vi "main.vi"() -> ()   [LabVIEW 2025]
uses:
  Controls/#typedef States.ctl
  Data.ctl
  <vilib>/Analysis/3filter.llb/Filter Passband Type.ctl
  <vilib>/sound2/lvsound2.llb/Sampling Mode.ctl
  <vilib>/sound2/lvsound2.llb/Sound Data Format.ctl
  <vilib>/Instr/_visa.llb/VISA Configure Serial Port (Instr).vi
  <vilib>/Analysis/3filter.llb/Butterworth Filter (DBL).vi
  <vilib>/sound2/lvsound2.llb/Sound Output Write (DBL Single).vi
  <vilib>/Analysis/NI_AALBase.lvlib
panel:
  in  "DETUNE":dbl(knob) scale=0.0..1.0
  out "zoom wave":dbl[](graph)
  in  "DRIVE":dbl(slide)=1.0 scale=0.5..5.0
  in  "NOTE":enum32{"BASS", "LOW MID", "MID", "HIGH", "LEAD"}(radio)
  in  "WAVE TYPE":u16(ring) items=["SIN", "SAW", "SQUARE", "TRIANGLE"]
  in  "PORT":refnum<visa-resource-name>
  in  "Sustain":dbl(knob) scale=0.001..1.0
  in  "CUTOFF":dbl(knob) scale=1000.0..10000.0
  in  "BITCRUSHER":dbl(knob) scale=1.0..50.0
  in  "Duration [sec]":dbl(slide) scale=0.1..1.0
  in  "Decay":dbl(knob) scale=0.0..1.0
  in  "Release":dbl(knob) scale=0.0..1.0
  in  "Attack":dbl(knob) scale=0.0..1.0
  out "synth wave":i8[](graph)
  in  "TEST":bool
  in  "TRACK":enum32{"Item 0", "Item 1", "", "  "}(radio)
  out "error out":errorcluster
  in  "error in (no error)":errorcluster
  in  "stop":bool
  in  "SEND":bool
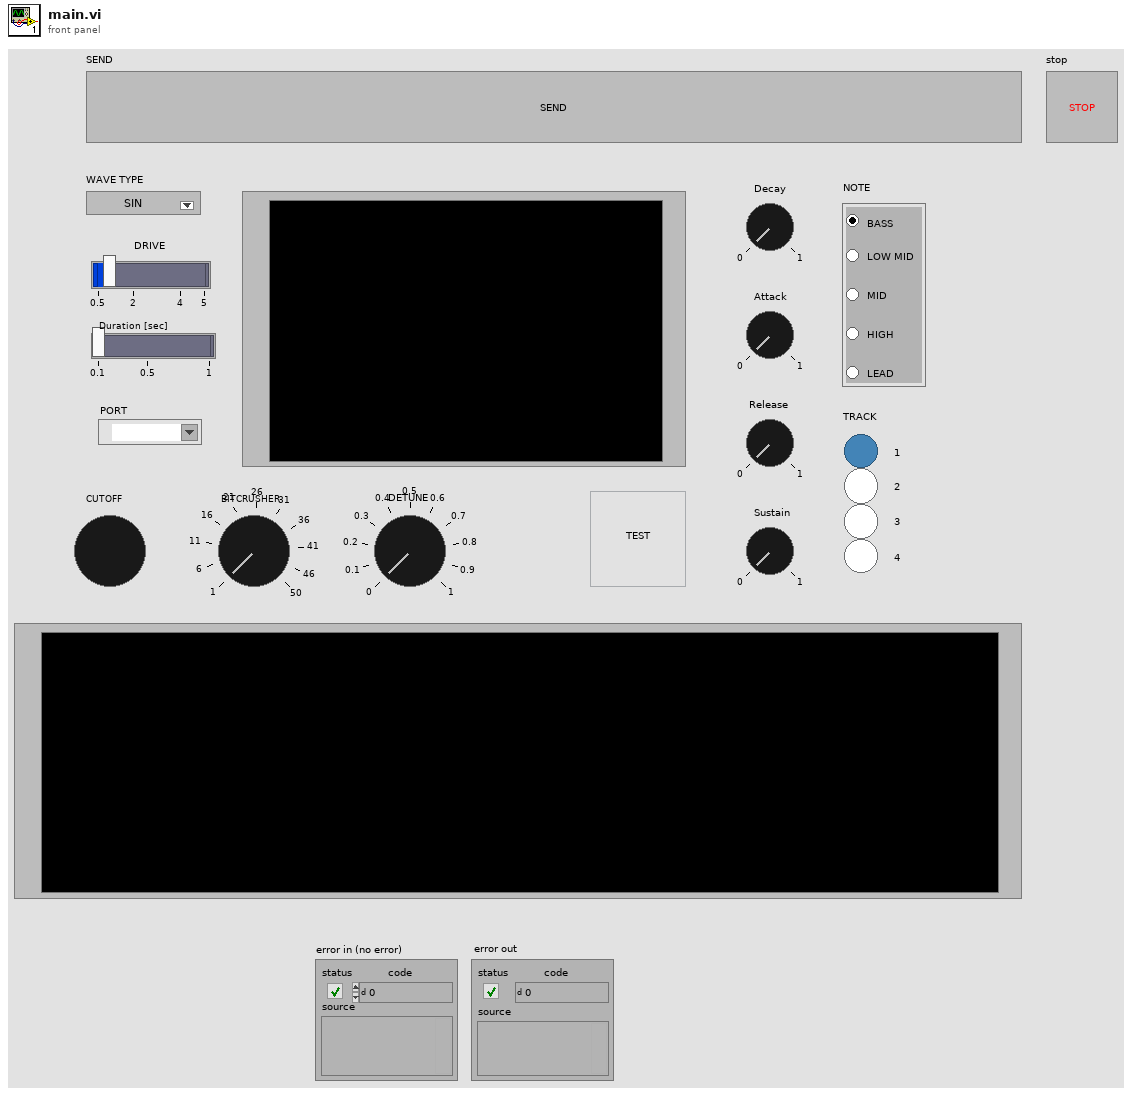
[diagram p1: front panel]
types:
  T1 = typedef "Data.ctl" = cluster{"Test/Send flag":bool, "TestData":dbl[], "8bitData":i8[], "VISA resource name":refnum<visa-resource-name>, "Decay":dbl, "Release":dbl, " Attack":dbl, "Sustain Level":dbl, "Cutoff":dbl, "Bitcrusher":dbl, "SampleLenght":dbl, "WAVE TYPE":u16, "Duration [sec]":dbl, "DRIVE":dbl, "NOTE":enum32{"BASS", "LOW MID", "MID", "HIGH", "LEAD"}, "Detune":dbl}
  T2 = typedef "#typedef States.ctl" = enum16{"Init", "Idle", "Generate", "Send", "Stop", "Test", "Error"}
  T3 = typedef "NI_AALBase.lvlib/Filter Passband Type.ctl" = enum32{"Lowpass", "Highpass", "Bandpass", "Bandstop"}
  T4 = typedef "Sound Data Format.ctl" = cluster{"sample rate (S/s)":dbl, "number of channels":i32, "bits per sample":i32}
  T5 = enum16{"Init", "Idle", "Generate", "Send", "Stop"}
  T6 = typedef "Sampling Mode.ctl" = i32
  T7 = typedef "Sound Output Task ID.ctl" = u32
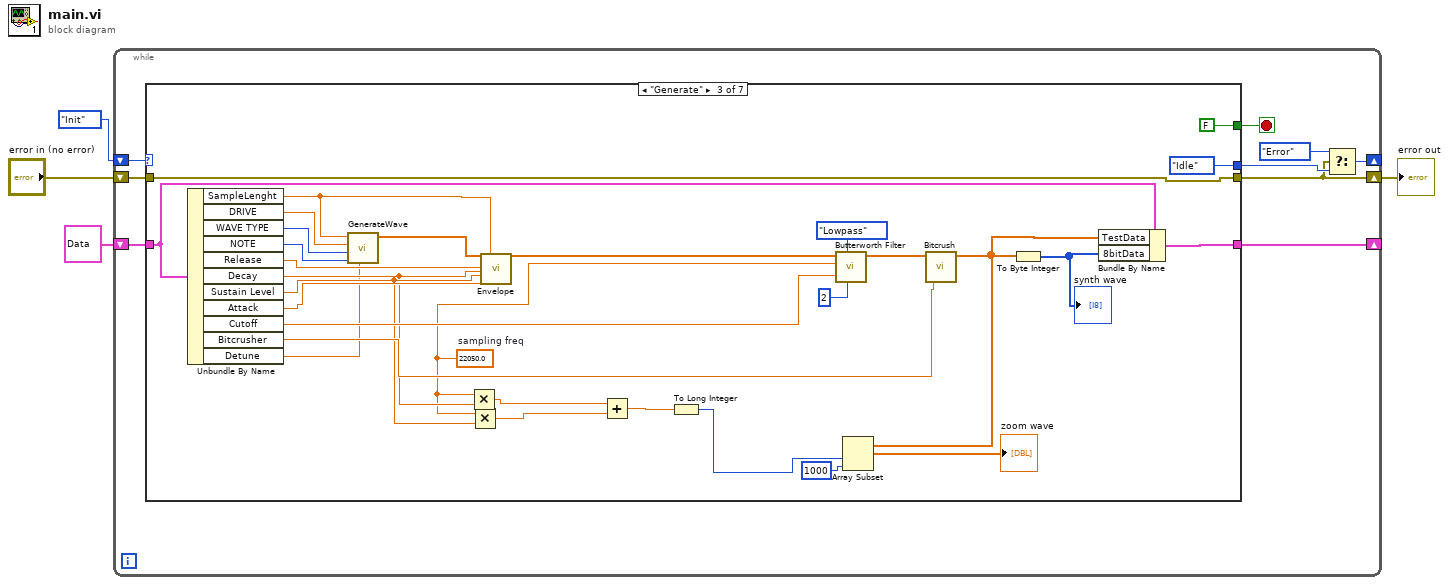
[diagram p0: block diagram]
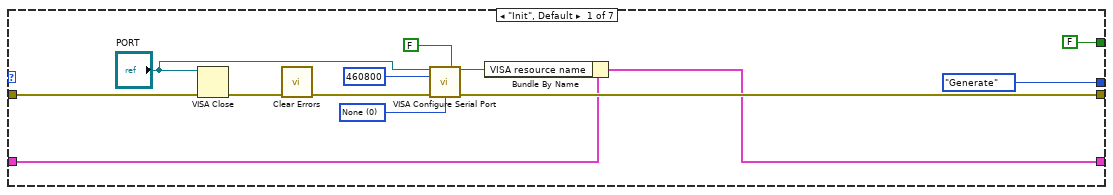
[diagram p2: hidden frame]
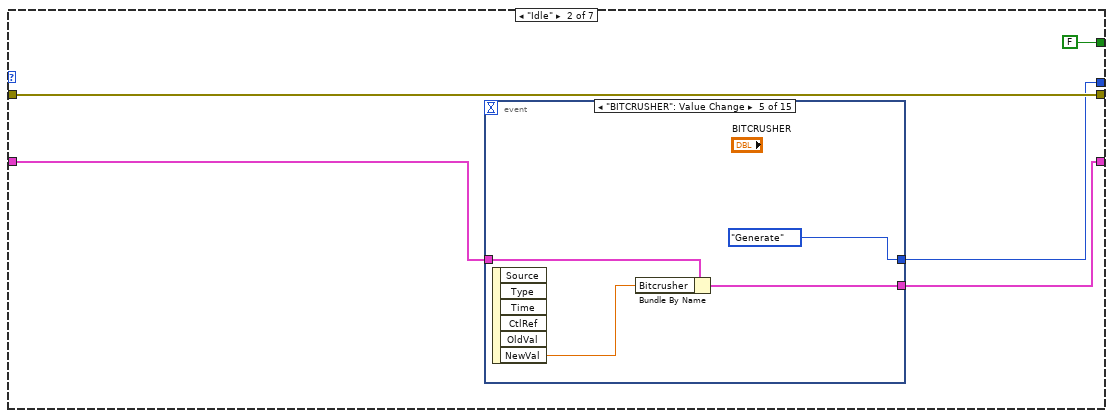
[diagram p3: hidden frame]
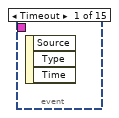
[diagram p4: hidden frame]
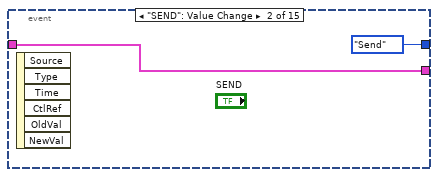
[diagram p5: hidden frame]
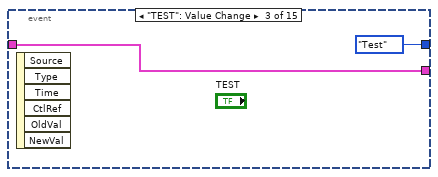
[diagram p6: hidden frame]
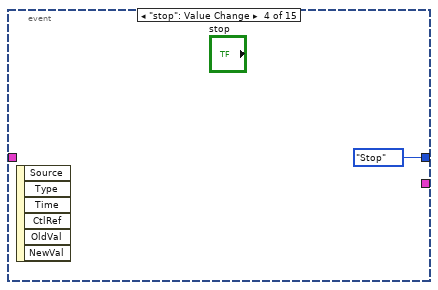
[diagram p7: hidden frame]
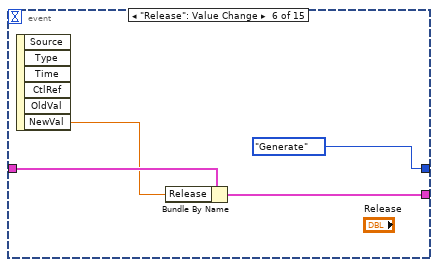
[diagram p8: hidden frame]
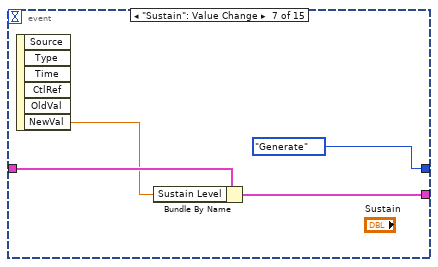
[diagram p9: hidden frame]
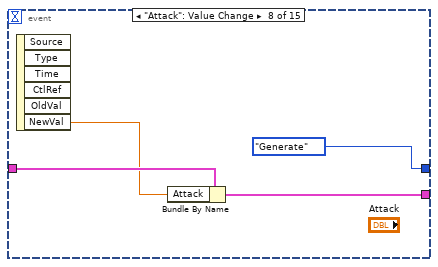
[diagram p10: hidden frame]
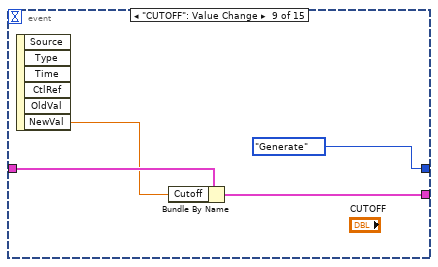
[diagram p11: hidden frame]
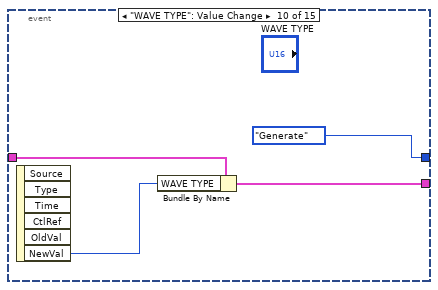
[diagram p12: hidden frame]
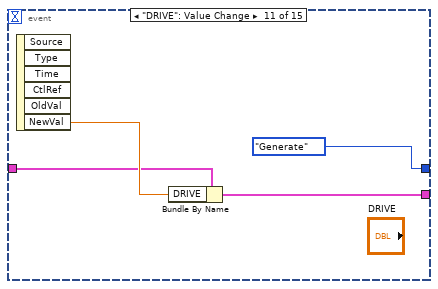
[diagram p13: hidden frame]
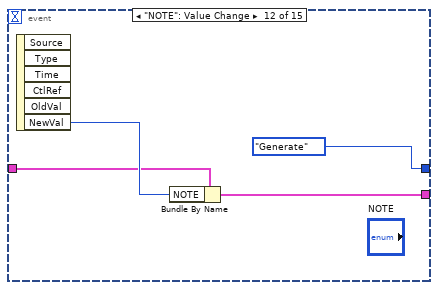
[diagram p14: hidden frame]
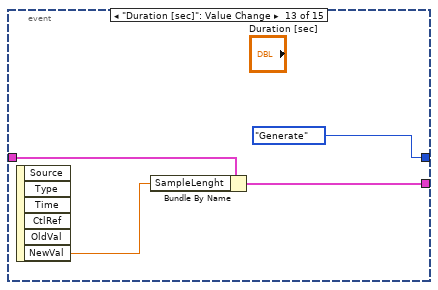
[diagram p15: hidden frame]
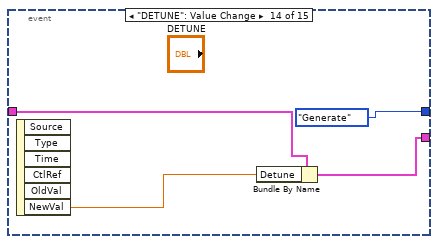
[diagram p16: hidden frame]
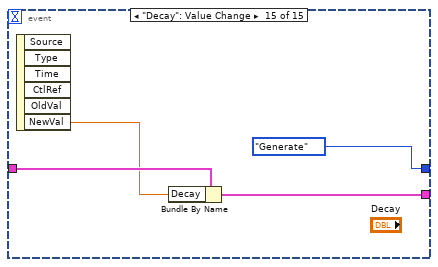
[diagram p17: hidden frame]
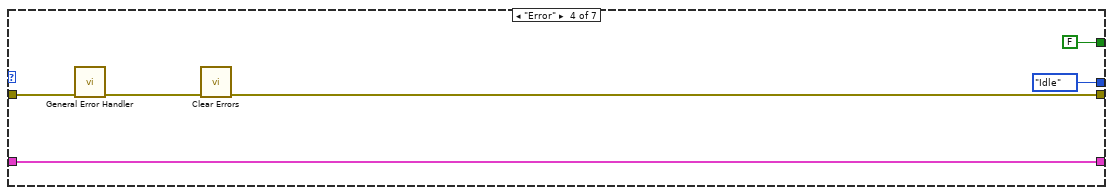
[diagram p18: hidden frame]
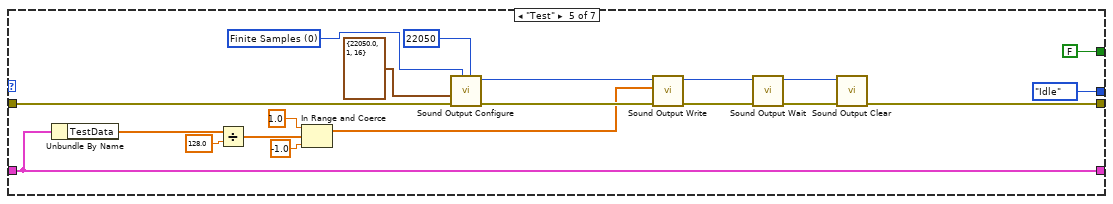
[diagram p19: hidden frame]
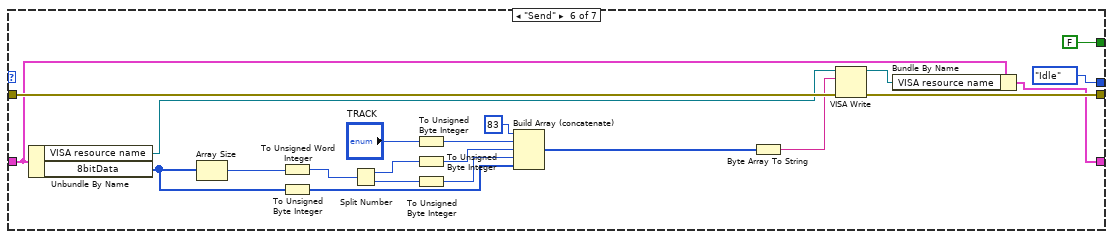
[diagram p20: hidden frame]
diagram:
  n1 = while {
    shift-right: [w6] -> _
    shift-left: #typedef_States."Init" -> [w13]
    shift-right: [w5] -> w2
    shift-left: "error in (no error)" -> [w12]
    shift-right: [w9] -> _
    shift-left: T1 {"Test/Send flag"=TRUE, "TestData"=[0.0], "8bitData"=[0], "VISA resource name"="", "Decay"=0.032, "Release"=0.1, " Attack"=0.08, "Sustain Level"=0.29, "Cutoff"=10000.0, "Bitcrusher"=1.0, "SampleLenght"=1.0, "WAVE TYPE"=0, "Duration [sec]"=1.0, "DRIVE"=1.009433962264151, "NOTE"=enum."BASS", "Detune"=0.0} ("Data") -> [w10]
    stop <- w11 stop-if-true
    n2 = case shown="\"Generate\"" w13 {
      tunnel: [w20 w31 w109 w114 w127 w153 w160] -> w5
      tunnel: w12 -> [w21 w31 w109 w116 w132 w154 w160]
      tunnel: [FALSE FALSE FALSE FALSE FALSE FALSE TRUE] -> w11
      tunnel: w10 -> [w18 w29 w103 w112 w125 w140 w159]
      tunnel: [w16 w28 w106 w112 w125 w138 w159] -> w9
      tunnel: [#typedef_States."Generate" w27 #typedef_States."Idle" #typedef_States."Idle" #typedef_States."Idle" #typedef_States."Idle" T5."Stop"] -> w7
      frame "Init", Default {
        w19 = u16 0 items=["None", "XON/XOFF", "RTS/CTS", "XON/XOFF & RTS/CTS", "DTR/DSR", "XON/XOFF & DTR/DSR"] ("flow control (0:none)")
        n3 = VISA Close(VISA resource name="PORT", error in (no error)=w21) -> (error out=w24:errorcluster)
        n4 = call <vilib>:"Clear Errors.vi"("error in (no error)"=w24) -> ("error out"=w23:errorcluster)  [unwired: 5 in, 1 out]
        n5 = call-poly "VISA Configure Serial Port"("VISA resource name"="PORT", "Enable Termination\nChar (T)"=FALSE ("Enable Termination\nChar (T)"), "baud rate (9600)"=u32 460800, "error in (no error)"=w23, "flow control (0:none)"=w19) -> ("VISA resource name out"=w17:refnum<visa-resource-name>, "error out"=w20:errorcluster)  [unwired: 9 in]
        n6 = Bundle By Name(cluster=w18, "VISA resource name"=w17) -> (w16:T1)
      }
      frame "Idle" {
        n7 = event shown="[4] \"BITCRUSHER\": Value Change" {
          selector: _ -> [_ _ _ _ _ _ _ _ _ _ _ _ _ _ _]
          dyn-events: _ -> [_ _ _ _ _ _ _ _ _ _ _ _ _ _ _]
          timeout: _ -> [_ _ _ _ _ _ _ _ _ _ _ _ _ _ _]
          tunnel: [_ #typedef_States."Send" #typedef_States."Test" #typedef_States."Stop" #typedef_States."Generate" #typedef_States."Generate" #typedef_States."Generate" #typedef_States."Generate" #typedef_States."Generate" #typedef_States."Generate" #typedef_States."Generate" #typedef_States."Generate" #typedef_States."Generate" #typedef_States."Generate" #typedef_States."Generate"] -> w27
          tunnel: w29 -> [_ w32 w34 _ w40 w44 w48 w52 w55 w60 w63 w67 w71 w74 w79]
          tunnel: [_ w32 w34 _ w39 w43 w47 w51 w54 w59 w62 w66 w70 w75 w78] -> w28
          event Timeout {
            n8 = event-data() -> ()  [unwired: 1 in, 3 out]
          }
          event "SEND": Value Change {
            n9 = event-data() -> ()  [unwired: 1 in, 6 out]
          }
          event "TEST": Value Change {
            n10 = event-data() -> ()  [unwired: 1 in, 6 out]
          }
          event "stop": Value Change {
            n11 = event-data() -> ()  [unwired: 1 in, 6 out]
          }
          event "BITCRUSHER": Value Change {
            n12 = event-data() -> ("NewVal"=w38:dbl)  [unwired: 1 in, 5 out]
            n13 = Bundle By Name(cluster=w40, "Bitcrusher"=w38) -> (w39:T1)
          }
          event "Release": Value Change {
            n14 = event-data() -> ("NewVal"=w41:dbl)  [unwired: 1 in, 5 out]
            n15 = Bundle By Name(cluster=w44, "Release"=w41) -> (w43:T1)
          }
          event "Sustain": Value Change {
            n16 = event-data() -> ("NewVal"=w45:dbl)  [unwired: 1 in, 5 out]
            n17 = Bundle By Name(cluster=w48, "Sustain Level"=w45) -> (w47:T1)
          }
          event "Attack": Value Change {
            n18 = event-data() -> ("NewVal"=w50:dbl)  [unwired: 1 in, 5 out]
            n19 = Bundle By Name(cluster=w52, "Attack"=w50) -> (w51:T1)
          }
          event "CUTOFF": Value Change {
            n20 = event-data() -> ("NewVal"=w53:dbl)  [unwired: 1 in, 5 out]
            n21 = Bundle By Name(cluster=w55, "Cutoff"=w53) -> (w54:T1)
          }
          event "WAVE TYPE": Value Change {
            n22 = event-data() -> ("NewVal"=w57:u16)  [unwired: 1 in, 5 out]
            n23 = Bundle By Name(cluster=w60, "WAVE TYPE"=w57) -> (w59:T1)
          }
          event "DRIVE": Value Change {
            n24 = event-data() -> ("NewVal"=w64:dbl)  [unwired: 1 in, 5 out]
            n25 = Bundle By Name(cluster=w63, "DRIVE"=w64) -> (w62:T1)
          }
          event "NOTE": Value Change {
            n26 = event-data() -> ("NewVal"=w68:enum32{"BASS", "LOW MID", "MID", "HIGH", "LEAD"})  [unwired: 1 in, 5 out]
            n27 = Bundle By Name(cluster=w67, "NOTE"=w68) -> (w66:T1)
          }
          event "Duration [sec]": Value Change {
            n28 = event-data() -> ("NewVal"=w72:dbl)  [unwired: 1 in, 5 out]
            n29 = Bundle By Name(cluster=w71, "SampleLenght"=w72) -> (w70:T1)
          }
          event "DETUNE": Value Change {
            n30 = event-data() -> ("NewVal"=w73:dbl)  [unwired: 1 in, 5 out]
            n31 = Bundle By Name(cluster=w74, "Detune"=w73) -> (w75:T1)
          }
          event "Decay": Value Change {
            n32 = event-data() -> ("NewVal"=w77:dbl)  [unwired: 1 in, 5 out]
            n33 = Bundle By Name(cluster=w79, "Decay"=w77) -> (w78:T1)
          }
        }
      }
      frame "Generate" {
        w86 = 22050.0  # sampling freq
        n34 = Unbundle By Name(w103) -> ("SampleLenght"=w98:dbl, "DRIVE"=w101:dbl, "WAVE TYPE"=w100:u16, "NOTE"=w99:enum32{"BASS", "LOW MID", "MID", "HIGH", "LEAD"}, "Release"=w97:dbl, "Decay"=w87:dbl, "Sustain Level"=w88:dbl, "Attack"=w96:dbl, "Cutoff"=w93:dbl, "Bitcrusher"=w92:dbl, "Detune"=w81:dbl)
        n35 = call "GenerateWave.vi"("Detune"=w81, "NOTE"=w99, "WAVE TYPE"=w100, "DRIVE"=w101, "SampleLenght"=w98) -> ("OUT"=w102:dbl[])  [unwired: 6 in]
        n36 = Multiply(x=w86, y=w87) -> (x*y=w85:dbl)
        n37 = Multiply(x=w86, y=w88) -> (x*y=w84:dbl)
        n38 = call "Envelope.vi"("IN"=w102, "Release"=w97, "Decay"=w87, "Sustain Level"=w88, "Attack"=w96, "SampleLenght"=w98) -> ("OUT"=w95:dbl[])  [unwired: 21 in]
        n39 = Add(x=w85, y=w84) -> (x+y=w83:dbl)
        n40 = To Long Integer(number=w83) -> (32bit integer=w82:i32)
        n41 = call-poly <vilib>:"Butterworth Filter.vi"("order"=2, "filter type"=Filter_Passband_Type."Lowpass", "low cutoff freq: fl"=w93, "sampling freq: fs"=w86, "X"=w95) -> ("Filtered X"=w94:dbl[])  [unwired: 3 in, 1 out]
        n42 = call "Bitcrush.vi"("IN"=w94, "Bitcrusher"=w92) -> ("OUT"=w90:dbl[])  [unwired: 7 in]
        n43 = Array Subset(array=w90, index=w82, length=1000) -> (→"zoom wave":dbl[])
        n44 = To Byte Integer(number=w90) -> (8bit integer=w105:i8[])
        "synth wave" <- w105
        n45 = Bundle By Name(cluster=w103, "TestData"=w90, "8bitData"=w105) -> (w106:T1)
      }
      frame "Error" {
        n46 = call <vilib>:"General Error Handler.vi"("error in (no error)"=w116) -> ("error out"=w115:errorcluster)  [unwired: 10 in, 4 out]
        n47 = call <vilib>:"Clear Errors.vi"("error in (no error)"=w115) -> ("error out"=w114:errorcluster)  [unwired: 5 in, 1 out]
      }
      frame "Test" {
        w136 = T6 0 items=["Finite Samples", "Continuous Samples"] ("sample mode")
        n48 = Unbundle By Name(w125) -> ("TestData"=w119:dbl[])
        n49 = Divide(x=w119, y=128.0) -> (x/y=w118:dbl[])
        n50 = In Range and Coerce(upper limit=1.0, x=w118, lower limit=-1.0) -> (coerced(x)=w120:dbl[])  [unwired: 1 out]
        n51 = call <vilib>:"Sound Output Configure.vi"("number of samples/ch"=22050, "sample mode"=w136, "error in (no error)"=w132, "sound format"=T4 {"sample rate (S/s)"=22050.0, "number of channels"=1, "bits per sample"=16}) -> ("error out"=w133:errorcluster, "task ID"=w134:T7)  [unwired: 6 in]
        n52 = call-poly <vilib>:"Sound Output Write.vi"("error in (no error)"=w133, "data"=w120, "task ID"=w134) -> ("error out"=w130:errorcluster, "task ID out"=w131:T7)  [unwired: 7 in]
        n53 = call <vilib>:"Sound Output Wait.vi"("error in (no error)"=w130, "task ID"=w131) -> ("error out"=w129:errorcluster, "task ID out"=w128:T7)  [unwired: 8 in]
        n54 = call <vilib>:"Sound Output Clear.vi"("error in (no error)"=w129, "task ID"=w128) -> ("error out"=w127:errorcluster)  [unwired: 9 in]
      }
      frame "Send" {
        n55 = Unbundle By Name(w140) -> ("VISA resource name"=w142:refnum<visa-resource-name>, "8bitData"=w141:i8[])
        n56 = Array Size(array=w141) -> (size(s)=w149:i32)
        n57 = To Unsigned Word Integer(number=w149) -> (unsigned 16bit integer=w143:u16)
        n58 = To Unsigned Byte Integer(number=w141) -> (unsigned 8bit integer=w150:u8[])
        n59 = Split Number(x=w143) -> (hi(x)=w148:u8, lo(x)=w147:u8)
        n60 = To Unsigned Byte Integer(number="TRACK") -> (unsigned 8bit integer=w151:u8)
        n61 = To Unsigned Byte Integer(number=w148) -> (unsigned 8bit integer=w146:u8)
        n62 = To Unsigned Byte Integer(number=w147) -> (unsigned 8bit integer=w145:u8)
        n63 = Build Array (concatenate)(u8 83, w151, w146, w145, w150) -> (w155:u8[])
        n64 = Byte Array To String(unsigned byte array=w155) -> (string=w144:string)
        n65 = VISA Write(VISA resource name=w142, write buffer=w144, error in (no error)=w154) -> (VISA resource name out=w139:refnum<visa-resource-name>, error out=w153:errorcluster)  [unwired: 1 out]
        n66 = Bundle By Name(cluster=w140, "VISA resource name"=w139) -> (w138:T1)
      }
      frame "Stop" {
      }
    }
    n67 = Select(t=#typedef_States."Error", s=w5, f=w7) -> (s? t:f=w6:T2)
  }
  "error out" <- w2
